vi "User32.GetDesktopWindow.vi"(11 "ErrorIn":errorcluster) -> (4 "DesktopHandle":i32, 15 "ErrorOut":errorcluster)   [LabVIEW 2021]
uses:
  user32.dll
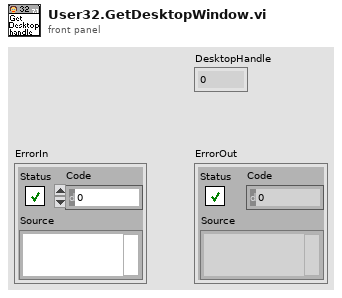
[diagram p1: front panel]
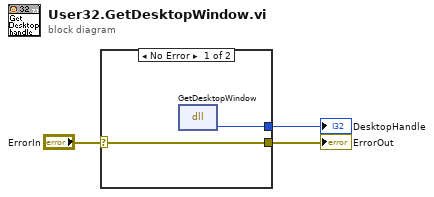
[diagram p0: block diagram]
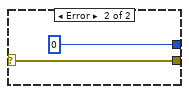
[diagram p2: hidden frame]
diagram:
  n1 = case shown="No Error" "ErrorIn" {
    selector: "ErrorIn" -> [w5 w7]
    tunnel: [w4 0] -> w1
    tunnel: [w5 w7] -> w2
    frame No Error {
      n2 = dll-call lib="user32.dll" fn="GetDesktopWindow"() -> (w4:i32)  [unwired: 3 in, 2 out]
    }
    frame Error {
    }
  }
  "DesktopHandle" <- w1
  "ErrorOut" <- w2
